vi "Grid KeyDown EnumCol.vi"(4 "表サイズ(縦×横)":i32[](array[numeric]), 6 "EditPos":T1, 8 "error in (no error)":errorcluster caption="エラー入力（エラーなし）", 9 "Char":i16, 10 "ref.表":refnum<vi>, 11 "Control入力":refnum<vi>) -> (0 "error out":errorcluster caption="エラー出力", 1 "セル文字列":string, 3 "ブール":bool)   [LabVIEW 2014]
uses:
  <vilib>/event_ctls.llb/eventvkey.ctl
  <vilib>/Utility/miscctls.llb/LVRowAndColumnTypeDef.ctl
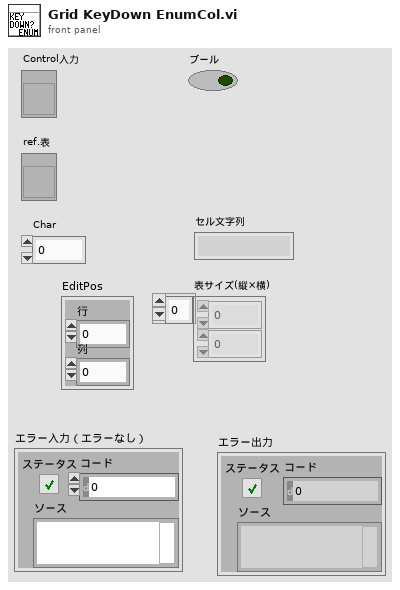
[diagram p1: front panel]
types:
  T1 = typedef "LVRowAndColumnTypeDef.ctl" = cluster{"Row":i32, "Column":i32}
  T2 = typedef "eventvkey.ctl" = enum16{"ASCII", "Enter", "Return", "Shift", "Ctrl", "Alt", "Cmd", "Opt", "Caps", "NumLock", "Clear", "Break", "Up", "Down", "Left", "Right", "Insert", "Delete", "Home", "End", "PageUp", "PageDown", "Escape", "Help", "Pause", "ScrollLock", "F1", "F2", "F3", "F4", "F5", "F6", "F7", "F8", "F9", "F10", "F11", "F12", "F13", "F14", "F15", "F16", "F17", "F18", "F19", "F20", "F21", "F22", "F23", "F24", "Play", "VolumeUp", "VolumeDown", "Mute", "Two Byte Char"}
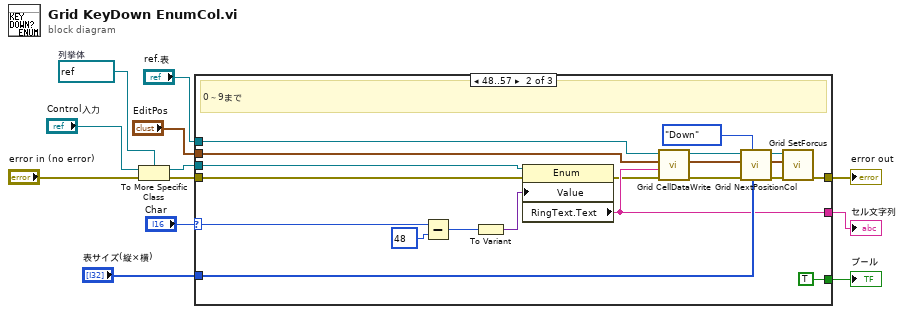
[diagram p0: block diagram]
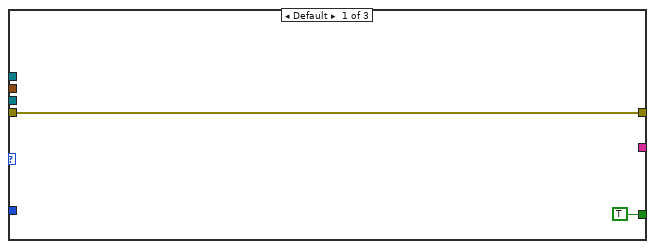
[diagram p2: hidden frame]
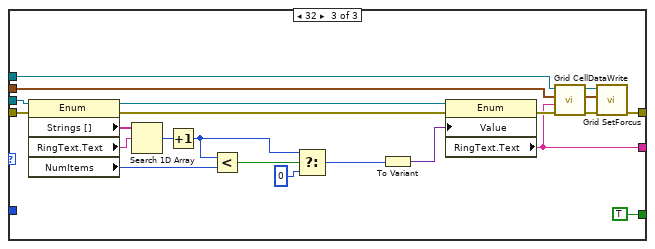
[diagram p3: hidden frame]
diagram:
  w6 = refnum<vi> refnum  # 列挙体
  n1 = To More Specific Class(target class=w6, reference="Control入力", error in="error in (no error)") -> (specific class reference=w8:refnum<vi>, error out=w2:errorcluster)
  n2 = case shown="48..57" "Char" {
    selector: "Char" -> [_ w34 _]
    tunnel: w8 -> [_ w30 w53]
    tunnel: "EditPos" -> [_ w23 w50]
    tunnel: "表サイズ(縦×横)" -> [_ w29 _]
    tunnel: [TRUE TRUE TRUE] -> w11
    tunnel: "ref.表" -> [_ w26 w51]
    tunnel: [_ w18 w35] -> w4
    tunnel: w2 -> [w13 w17 w38]
    tunnel: [w13 w15 w36] -> w1
    frame Default {
    }
    frame 48..57 {
      # "0～9まで"
      n3 = Subtract(x=w34, y=i16 48) -> (x-y=w32:i16)
      n4 = To Variant(anything=w32) -> (Variant=w31:variant)
      n5 = property class="Enum"(reference=w30, error in=w17, "Value"=w31) -> (error out=w16:errorcluster, "RingText.Text"=w18:string)  [unwired: 1 out]
      n6 = call "Grid CellDataWrite.vi"("error in (no error)"=w16, "RingText.Text"=w18, "EditPos"=w23, "Table入力"=w26) -> ("エラー出力"=w20:errorcluster, "EditPos(copy))"=w22:T1, "Table出力"=w25:refnum<vi>)  [unwired: 5 in]
      n7 = call "Grid NextPositionCol.vi"("表サイズ(縦x横)"=w29, "VKey(Right)"=eventvkey."Down" ("VKey"), "error in (no error)"=w20, "EditPos入力"=w22, "ref.表"=w25) -> ("error out"=w19:errorcluster, "EditPos出力"=w21:T1, "ref.表(copy)"=w24:refnum<vi>)  [unwired: 4 in]
      n8 = call "Grid SetForcus.vi"("エラー入力（エラーなし）"=w19, "EditPos入力"=w21, "Table入力"=w24) -> ("error out"=w15:errorcluster)  [unwired: 6 in, 2 out]
    }
    frame 32 {
      n9 = property class="Enum"(reference=w53, error in=w38) -> (reference out=w42:refnum<vi>, error out=w39:errorcluster, "Strings []"=w46:string[], "RingText.Text"=w45:string, "NumItems"=w43:u32)
      n10 = Search 1D Array(1D array=w46, element=w45) -> (index of element=w44:i32)  [unwired: 1 in]
      n11 = Increment(x=w44) -> (x+1=w40:i32)
      n12 = Less?(x=w40, y=w43) -> (x < y?=w56:bool)
      n13 = Select(t=w40, s=w56, f=u16 0) -> (s? t:f=w55:i32)
      n14 = To Variant(anything=w55) -> (Variant=w54:variant)
      n15 = property class="Enum"(reference=w42, error in=w39, "Value"=w54) -> (error out=w37:errorcluster, "RingText.Text"=w35:string)  [unwired: 1 out]
      n16 = call "Grid CellDataWrite.vi"("error in (no error)"=w37, "RingText.Text"=w35, "EditPos"=w50, "Table入力"=w51) -> ("エラー出力"=w47:errorcluster, "EditPos(copy))"=w48:T1, "Table出力"=w49:refnum<vi>)  [unwired: 5 in]
      n17 = call "Grid SetForcus.vi"("エラー入力（エラーなし）"=w47, "EditPos入力"=w48, "Table入力"=w49) -> ("error out"=w36:errorcluster)  [unwired: 6 in, 2 out]
    }
  }
  "ブール" <- w11
  "error out" <- w1
  "セル文字列" <- w4
